vi "搜索字符串.vi"() -> (1 "起始位置":string[](array[string]), 2 "终止位置":string[](array[string]))   [LabVIEW 2018]
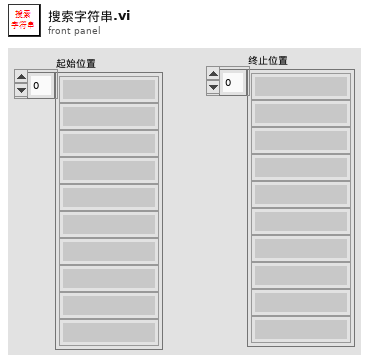
[diagram p1: front panel]
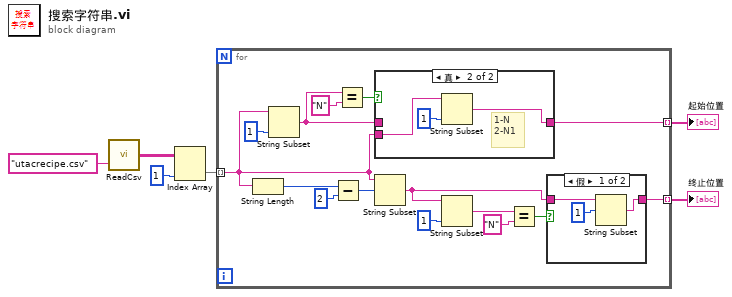
[diagram p0: block diagram]
diagram:
  n1 = call "ReadCsv.vi"("相对路径"="utacrecipe.csv") -> ("all rows"=w3:string[][])  [unwired: 1 in]
  n2 = Index Array(array=w3, index (col)=1 ("禁用的索引 (列)")) -> (element=w1:string[])  [unwired: 1 in]
  n3 = for {
    tunnel: w1 -> [w16] mode=indexing
    tunnel: [w17] -> w6 mode=indexing
    tunnel: [w7] -> w5 mode=indexing
    n4 = String Length(string=w16) -> (length=w15:i32)
    n5 = String Subset(string=w16, length (rest)=1 ("长度（剩余）")) -> (substring=w18:string)  [unwired: 1 in]
    n6 = Subtract(x=w15, y=2) -> (x-y=w13:i32)
    n7 = Equal?(x=w18, y="N") -> (x = y?=w20:bool)
    n8 = case shown="真" w20 {
      tunnel: w18 -> [w26 _]
      tunnel: [w26 w27] -> w17
      tunnel: w16 -> [_ w29]
      frame False {
      }
      frame True {
        # "1-N\n2-N1"
        n9 = String Subset(string=w29, length (rest)=1 ("长度（剩余）")) -> (substring=w27:string)  [unwired: 1 in]
      }
    }
    n10 = String Subset(string=w16, offset (0)=w13) -> (substring=w8:string)  [unwired: 1 in]
    n11 = String Subset(string=w8, length (rest)=1 ("长度（剩余）")) -> (substring=w9:string)  [unwired: 1 in]
    n12 = Equal?(x=w9, y="N") -> (x = y?=w11:bool)
    n13 = case shown="假" w11 {
      tunnel: w8 -> [w24 w25]
      tunnel: [w22 w25] -> w7
      frame False {
        n14 = String Subset(string=w24, offset (0)=1 ("偏移量(0)")) -> (substring=w22:string)  [unwired: 1 in]
      }
      frame True {
      }
    }
  }
  "起始位置" <- w6
  "终止位置" <- w5
